vi "DriveForDistancePID.vi"(8 "error in (no error)":errorcluster, 9 "RobotDriveRef":T1={"RobotDriveDevRef"={"DevStatus"={"status"=FALSE, "code"=0, "source"=""}, "Motors[]"=[], "Square Inputs"=FALSE, "Max Output"=0.0}, "Control Mode"=enum."Percent VBus", "Motor Settings"={"Wheel Radius"=0.0, "Encoder Ticks Per Rev"=0.0, "Gear Ratio"=0.0, "ClimbRev"=0.0}, "Default Control Mode"=enum."Unchanged / Invalid"}, 10 "SubSystem Data":T10, 11 "Command Loop Data":cluster{"Start Time (ms)":u32, "Iterations":i32}) -> (0 "error out":errorcluster, 1 "RobotDriveRef Out":T1={"RobotDriveDevRef"={"DevStatus"={"status"=FALSE, "code"=0, "source"=""}, "Motors[]"=[], "Square Inputs"=FALSE, "Max Output"=0.0}, "Control Mode"=enum."Percent VBus", "Motor Settings"={"Wheel Radius"=0.0, "Encoder Ticks Per Rev"=0.0, "Gear Ratio"=0.0, "ClimbRev"=0.0}, "Default Control Mode"=enum."Unchanged / Invalid"}, 2 "Finished":bool, 3 "Left Setpoint":dbl, 4 "Wait Time":dbl)   [LabVIEW 2015]
uses:
  Drive Setpoints.ctl
  Drive Operations.ctl
  Advanced Drive VIs/RobotDrive Type Def.ctl
  <vilib>/Rock Robotics/WPI/MotorControl/WPI_MotorControlDeviceRef.ctl
  <vilib>/Rock Robotics/WPI/MotorControl/WPI_MotorControlType.ctl
  <vilib>/Rock Robotics/SystemInterfaces/DIO/FPGA_DIOPWMChannel.ctl
  <vilib>/Rock Robotics/WPI/PWM/WPI_PWMDeadband.ctl
  <vilib>/Rock Robotics/WPI/CAN/Jaguar/SubVIs/WPI_CANJaguar_ControlMode.ctl
  <vilib>/Rock Robotics/WPI/CAN/TalonSRX/WPI_CANTalonSRX_APIControlMode.ctl
  Advanced Drive VIs/Drive Motor Settings.ctl
  <vilib>/addons/control/pid/pid.llb/PID (DBL).vi
  <vilib>/addons/control/pid/NI_PID_pid.lvlib
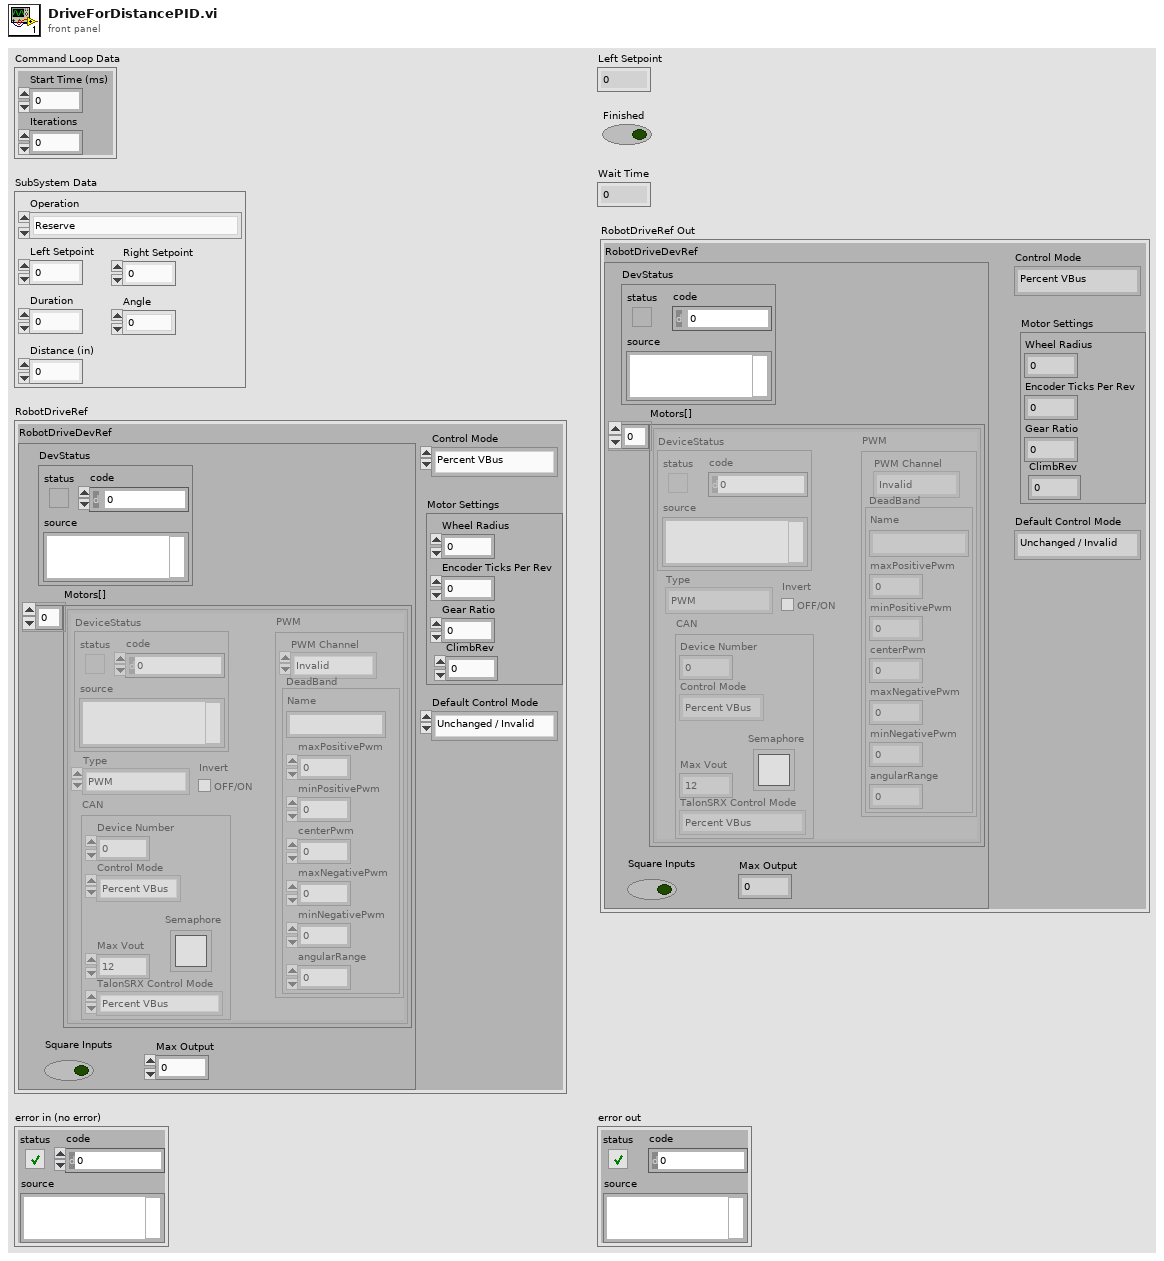
[diagram p1: front panel]
types:
  T1 = typedef "RobotDrive Type Def.ctl" = cluster{"RobotDriveDevRef":cluster{"DevStatus":errorcluster, "Motors[]":T2[], "Square Inputs":bool, "Max Output":dbl}, "Control Mode":T8, "Motor Settings":T9, "Default Control Mode":T8}
  T2 = typedef "WPI_MotorControlDeviceRef.ctl" = cluster{"DeviceStatus":errorcluster, "Type":T3, "PWM":cluster{"PWM Channel":T4, "DeadBand":T5}, "CAN":cluster{"Device Number":u8, "Control Mode":T6, "Semaphore":T7, "Max Vout":dbl, "TalonSRX Control Mode":T8}, "Invert":bool}
  T3 = typedef "WPI_MotorControlType.ctl" = enum16{"PWM", "CAN", "CANTalonSRX"}
  T4 = typedef "FPGA_DIOPWMChannel.ctl" = enum8{"PWM 0", "PWM 1", "PWM 2", "PWM 3", "PWM 4", "PWM 5", "PWM 6", "PWM 7", "PWM 8", "PWM 9", "PWM MXP 0", "PWM MXP 1", "PWM MXP 2", "PWM MXP 3", "PWM MXP 4", "PWM MXP 5", "PWM MXP 6", "PWM MXP 7", "PWM MXP 8", "PWM MXP 9", "Invalid"}
  T5 = typedef "WPI_PWMDeadband.ctl" = cluster{"Name":string, "maxPositivePwm":i32, "minPositivePwm":i32, "centerPwm":i32, "maxNegativePwm":i32, "minNegativePwm":i32, "angularRange":u16}
  T6 = typedef "WPI_CANJaguar_ControlMode.ctl" = enum8{"Percent VBus", "Current", "Speed", "Position", "Voltage"}
  T7 = typedef "Semaphore RefNum" = refnum<k1>
  T8 = typedef "WPI_CANTalonSRX_APIControlMode.ctl" = enum8{"Percent VBus", "Speed", "Position", "Slave", "Unchanged / Invalid", "Voltage Compensation", "Current", "Motion Profile"}
  T9 = typedef "Drive Motor Settings.ctl" = cluster{"Wheel Radius":dbl, "Encoder Ticks Per Rev":dbl, "Gear Ratio":dbl, "ClimbRev":dbl}
  T10 = typedef "Drive Setpoints.ctl" = cluster{"Operation":T11, "Left Setpoint":dbl, "Right Setpoint":dbl, "Duration":dbl, "Angle":dbl, "Distance (in)":dbl}
  T11 = typedef "Drive Operations.ctl" = enum16{"Reserve", "Read Current", "Immediate", "Drive for Time", "Drive for Distance", "Turn Degrees"}
  T12 = cluster{"proportional gain (Kc)":dbl, "integral time (Ti, min)":dbl, "derivative time (Td, min)":dbl}
  T13 = typedef "WPI_CANTalonSRX_GlobalStatus.ctl" = cluster{"Applied Throttle":dbl, "Module Enabled":bool, "CAN Error":errorcluster, "Closed Loop Error":dbl, "Forward Limit Switch Closed":bool, "Reverse Limit Switch Closed":bool, "Sensor Position":dbl, "Sensor Velocity":dbl, "Current":dbl, "Sticky Fault - Over Temp":bool, "Sticky Fault - Under Voltage":bool, "Sticky Fault - Forward Limit":bool, "Sticky Fault - Reverse Limit":bool, "Sticky Fault - Forward Soft Limit":bool, "Sticky Fault - Reverse Soft Limit":bool, "Brake is Enabled":bool, "Encoder Position":dbl, "Encoder Velocity":dbl, "Encoder Index Count":dbl, "Encoder A Pin State":bool, "Encoder B Pin State":bool, "Encoder Index Pin State":bool, "Analog In":dbl, "Analog In Velocity":dbl, "Temperature (C)":dbl, "Battery Voltage":dbl, "Control 5 Is Supported":bool, "Current Profile Slot Select":dbl, "Pos Div 8":bool, "Vel Div 4":bool, "Pulse Width Position":i32, "Pulse Width Velocity":i32, "Pulse Width Rise To Rise (us)":i32, "Pulse Width Rise To Fall (us)":i32, "Mot Prof Active Is Under Run":bool, "Mot Prof Active Has Under Run":bool, "Mot Prof Active Is Last":bool, "Mot Prof Active Velocity Only":bool, "Mot Prof Active Is Valid":bool, "Mot Prof Buffer Is Full":bool, "Mot Prof Active Profile Slot Select":i32, "Mot Prof NextID":i32, "Mot Prof Count":i32, "Mot Prof Active Velocity":dbl, "Mot Prof Active Position":dbl, "Mot Prof Output Enable":i32}
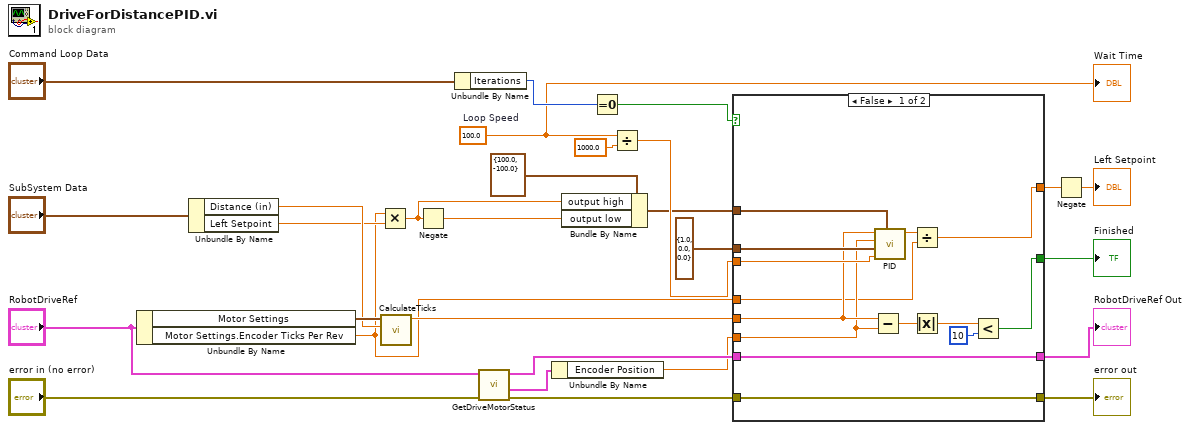
[diagram p0: block diagram]
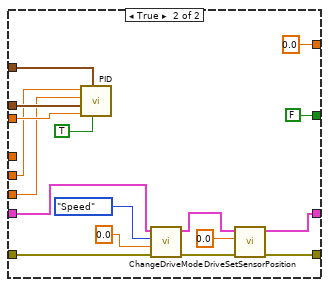
[diagram p2: hidden frame]
diagram:
  w18 = 100.0  # Loop Speed
  n1 = Unbundle By Name("RobotDriveRef") -> ("Motor Settings"=w14:T9, "Motor Settings.Encoder Ticks Per Rev"=w2:dbl)
  n2 = Unbundle By Name("SubSystem Data") -> ("Distance (in)"=w6:dbl, "Left Setpoint"=w5:dbl)
  n3 = Multiply(x=w2, y=w5) -> (x*y=w4:dbl)
  n4 = call "CalculateTicks.vi"("Distance (in)"=w6, "Motor Settings"=w14) -> ("Ticks"=w13:dbl)  [unwired: 9 in]
  n5 = Negate(x=w4) -> (-x=w15:dbl)
  n6 = Unbundle By Name("Command Loop Data") -> ("Iterations"=w26:i32)
  n7 = call "GetDriveMotorStatus.vi"("error in (no error)"="error in (no error)", "RobotDriveRef In"="RobotDriveRef") -> ("error out"=w9:errorcluster, "Right"=w1:T13, "RobotDriveRef Out"=w7:T1)  [unwired: 6 in, 1 out]
  n8 = Unbundle By Name(w1) -> ("Encoder Position"=w3:dbl)
  n9 = Bundle By Name(cluster=cluster{"output high":dbl, "output low":dbl} {"output high"=100.0, "output low"=-100.0} ("output range"), "output high"=w4, "output low"=w15) -> (w12:cluster{"output high":dbl, "output low":dbl})
  n10 = Equal To 0?(x=w26) -> (x = 0?=w25:bool)
  n11 = Divide(x=w18, y=1000.0) -> (x/y=w17:dbl)
  n12 = case shown="False" w25 {
    tunnel: [w37 FALSE ("ignore previous (F)")] -> w23
    tunnel: [w29 0.0 ("output")] -> w22
    tunnel: [w34 w53] -> w27
    tunnel: T12 {"proportional gain (Kc)"=1.0, "integral time (Ti, min)"=0.0, "derivative time (Td, min)"=0.0} ("PID gains") -> [w42 w50]
    tunnel: w17 -> [w41 w51]
    tunnel: w13 -> [w36 w48]
    tunnel: w12 -> [w35 w49]
    tunnel: w9 -> [w33 w47]
    tunnel: [w33 w46] -> w8
    tunnel: w7 -> [w34 w43]
    tunnel: w3 -> [w32 w45]
    tunnel: w2 -> [w31 _]
    frame False {
      n13 = Subtract(x=w36, y=w32) -> (x-y=w40:dbl)
      n14 = call-poly <vilib>:"PID.vi"("output range"=w35, "dt (s)"=w41, "PID gains"=w42, "process variable"=w32, "setpoint"=w36) -> ("output"=w30:dbl)  [unwired: 5 in, 1 out]
      n15 = Divide(x=w30, y=w31) -> (x/y=w29:dbl)
      n16 = Absolute Value(x=w40) -> (abs(x)=w39:dbl)
      n17 = Less?(x=w39, y=10) -> (x < y?=w37:bool)
    }
    frame True {
      n18 = call-poly <vilib>:"PID.vi"("reinitialize? (F)"=TRUE, "output range"=w49, "dt (s)"=w51, "PID gains"=w50, "process variable"=w45, "setpoint"=w48) -> ()  [unwired: 4 in, 2 out]
      n19 = call "ChangeDriveMode.vi"("error in (no error)"=w47, "Output"=0.0, "Control Mode"=WPI_CANTalonSRX_APIControlMode."Speed", "RobotDriveRef"=w43) -> ("error out"=w56:errorcluster, "RobotDriveRef Out"=w57:T1)  [unwired: 6 in]
      n20 = call "DriveSetSensorPosition.vi"("error in (no error)"=w56, "New Sensor Position"=0.0, "RobotDriveRef In"=w57) -> ("error out"=w46:errorcluster, "RobotDriveRef Out"=w53:T1)  [unwired: 7 in]
    }
  }
  "error out" <- w8
  "RobotDriveRef Out" <- w27
  "Finished" <- w23
  n21 = Negate(x=w22) -> (-x=→"Left Setpoint":dbl)
  "Wait Time" <- w18
